vi "MSScript_SubVI_ExtractSelectedString.vi"(5 "Selections":cluster{"Start":u32, "End":u32}[](array[cluster]), 6 "Selection bias":u32, 7 "String in":string="str") -> (2 "Non selected string":string, 3 "Selected strings":string[](array[string]))   [LabVIEW 2018, in "MSScript.lvclass"]
uses:
  MSScript.lvclass
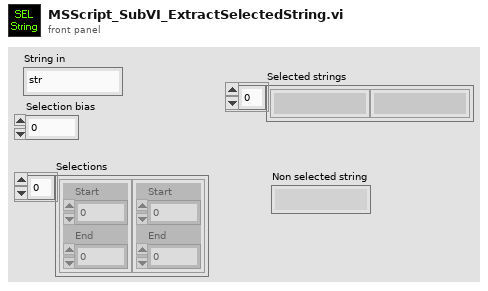
[diagram p1: front panel]
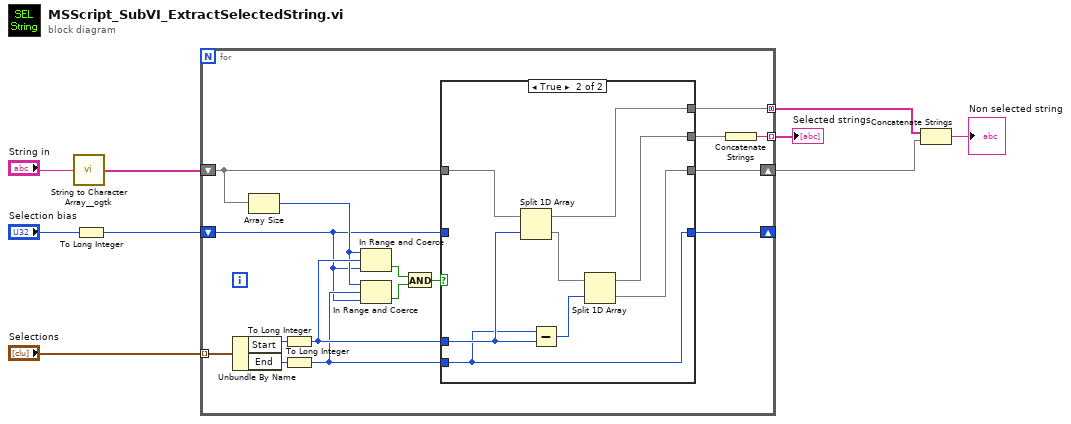
[diagram p0: block diagram]
diagram:
  n1 = call <userlib>:"String to Character Array__ogtk.vi"("Input String"="String in") -> ("Character Array"=w6:string[])
  n2 = To Long Integer(number="Selection bias") -> (32bit integer=w5:i32)
  n3 = for {
    tunnel: "Selections" -> [w25] mode=indexing
    shift-right: [w14] -> w2
    shift-left: w6 -> [w17]
    shift-right: [w15] -> _
    shift-left: w5 -> [w13]
    tunnel: [w12] -> w3 mode=concatenating
    tunnel: [w10] -> w4 mode=indexing
    n4 = Unbundle By Name(w25) -> ("Start"=w24:u32, "End"=w23:u32)
    n5 = Array Size(array=w17) -> (size(s)=w16:i32)
    n6 = To Long Integer(number=w24) -> (32bit integer=w19:i32)
    n7 = To Long Integer(number=w23) -> (32bit integer=w18:i32)
    n8 = In Range and Coerce(upper limit=w16, x=w19, lower limit=w13) -> (In Range?=w22:bool)  [unwired: 1 out]
    n9 = In Range and Coerce(upper limit=w16, x=w18, lower limit=w13) -> (In Range?=w21:bool)  [unwired: 1 out]
    n10 = And(x=w22, y=w21) -> (x .and. y?=w20:bool)
    n11 = case shown="True" w20 {
      tunnel: w19 -> [_ w34]
      tunnel: w18 -> [_ w30]
      tunnel: w17 -> [w27 w35]
      tunnel: [w26 w30] -> w15
      tunnel: [w27 w31] -> w14
      tunnel: w13 -> [w26 _]
      tunnel: [_ w29] -> w12
      tunnel: [_ w28] -> w11
      frame False {
      }
      frame True {
        n12 = Split 1D Array(array=w35, index=w34) -> (first subarray=w29:string[], second subarray=w32:string[])
        n13 = Subtract(x=w30, y=w34) -> (x-y=w33:i32)
        n14 = Split 1D Array(array=w32, index=w33) -> (first subarray=w28:string[], second subarray=w31:string[])
      }
    }
    n15 = Concatenate Strings(w11) -> (w10:string)
  }
  "Selected strings" <- w4
  n16 = Concatenate Strings(w3, w2) -> (→"Non selected string":string)
